vi "Deallocate refnums.vi"(8 "error in (no error)":errorcluster, 11 "TDCHits Buffer":T1) -> (0 "error out":errorcluster)   [LabVIEW 2016, in "HPTDC Driver Library.lvlib"]
uses:
  HPTDC Driver Library.lvlib
  Typedefs/TDCHitObjBuffer.ctl
  C:/Users/CRT Controller/CRTC Labview Application/Source/HPTDC Driver Library Folder/Library files/hptdc_net4_3.7.0_x64.dll
  hptdc_net4_3.7.0_x64.dll
  VIs/Global Variables/System info.vi
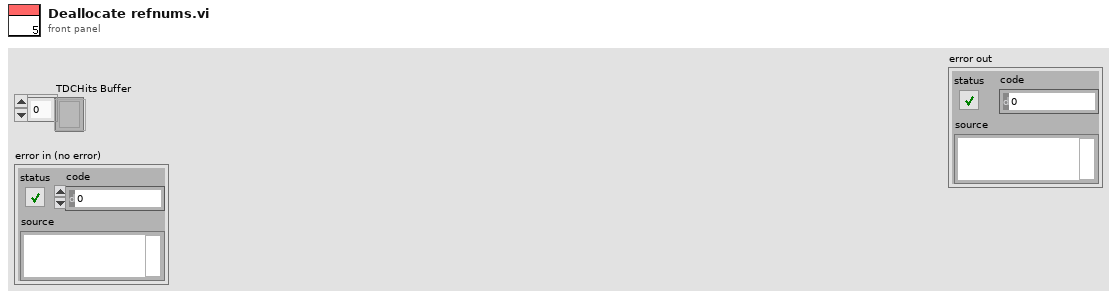
[diagram p1: front panel]
types:
  T1 = typedef "TDCHitObjBuffer.ctl" = refnum<k24>[]
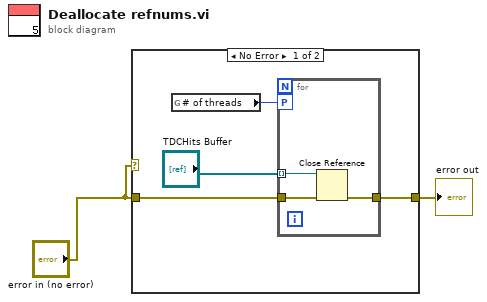
[diagram p0: block diagram]
diagram:
  n1 = case shown="No Error" "error in (no error)" {
    tunnel: "error in (no error)" -> [w5 w10]
    tunnel: [w4 w10] -> w2
    frame No Error {
      n2 = global read "System info.vi" "# of threads"() -> (w3:i32)
      n3 = for {
        tunnel: "TDCHits Buffer" -> [w9] mode=indexing
        workers-P: w3 -> [_]
        tunnel: w5 -> [w7]
        tunnel: [w8] -> w4
        n4 = Close Reference(reference=w9, error in (no error)=w7) -> (error out=w8:errorcluster)
      }
    }
    frame Error {
    }
  }
  "error out" <- w2
